vi "Initialize.vi"(2 "XRef":refnum<vi>) -> (1 "State Out":T1)   [LabVIEW 2012, in "ArrayDimension.xnode"]
uses:
  ArrayDimension.xnode
  State.ctl
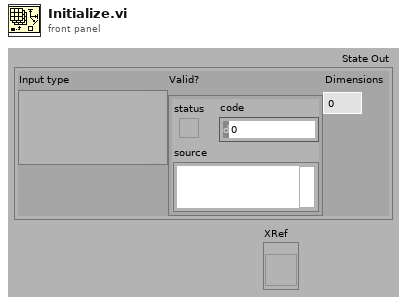
[diagram p1: front panel]
types:
  T1 = typedef "ArrayDimension.xnode/State.ctl" = cluster{"Input type":variant, "Valid?":errorcluster, "Dimensions":i32}
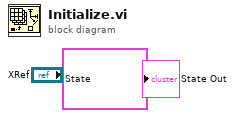
[diagram p0: block diagram]
diagram:
  "State Out" <- T1 {"Input type"=variant, "Valid?"={"status"=TRUE, "code"=0, "source"="Initialised"}, "Dimensions"=0} ("State Out")
